vi "Get Category Summaries.vi"(8 "error in (no error)":errorcluster, 9 "Month":T1, 10 "YYYY":i32, 11 "Database in":refnum<class "Account History.lvclass">) -> (0 "error out":errorcluster, 2 "Category Summaries":refnum<class "Expense Summary.lvclass">[](array[class]), 3 "Database out":refnum<class "Account History.lvclass">)   [LabVIEW 2018, in "Account History.lvclass"]
uses:
  Account History.lvclass
  Expense Summary/Expense Summary.lvclass
  Month.ctl
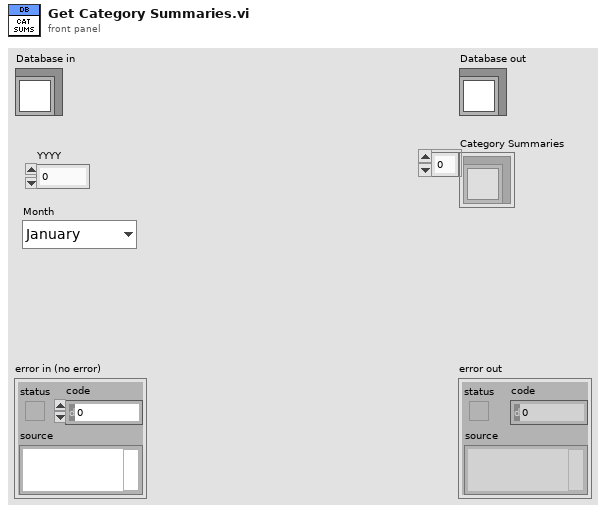
[diagram p1: front panel]
types:
  T1 = typedef "Account History.lvclass/Month.ctl" = enum16{"January", "February", "March", "April", "May", "June", "July", "August", "September", "October", "November", "December"}
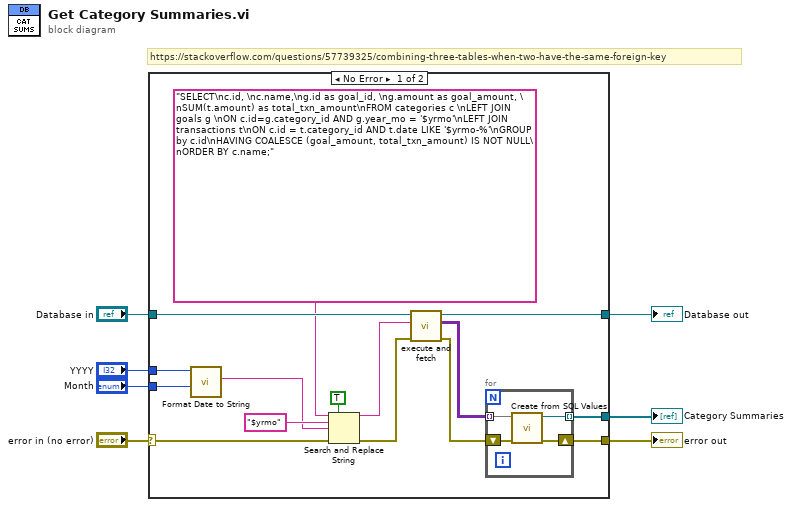
[diagram p0: block diagram]
diagram:
  # "https://stackoverflow.com/questions/57739325/combining-three-tables-when-two-have-the-same-foreign-key"
  n1 = case shown="No Error" "error in (no error)" {
    selector: "error in (no error)" -> [w17 w27]
    tunnel: [w20 w28] -> w7
    tunnel: "Database in" -> [w19 w28]
    tunnel: [w18 w27] -> w5
    tunnel: [w11 _] -> w3
    tunnel: "YYYY" -> [w9 _]
    tunnel: "Month" -> [w8 _]
    frame No Error {
      n2 = call "Format Date to String.vi"("Month"=w8, "YYYY"=w9) -> ("Year-Mo"=w10:string)  [unwired: 9 in]
      n3 = Search and Replace String(replace all?=TRUE ("replace all? (F)"), input string="SELECT\nc.id, \nc.name,\ng.id as goal_id, \ng.amount as goal_amount, \nSUM(t.amount) as total_txn_amount\nFROM categories c \nLEFT JOIN goals g \nON c.id=g.category_id AND g.year_mo = '$yrmo'\nLEFT JOIN transactions t\nON c.id = t.category_id AND t.date LIKE '$yrmo-%'\nGROUP by c.id\nHAVING COALESCE (goal_amount, total_txn_amount) IS NOT NULL\nORDER BY c.name;", search string="$yrmo", replace string=w10, error in=w17) -> (result string=w12:string, error out=w13:errorcluster)  [unwired: 3 in, 2 out]
      n4 = call "execute and fetch.vi"("error in (no error)"=w13, "SQL query"=w12, "Database in"=w19) -> ("error out"=w21:errorcluster, "recordset data"=w22:variant[][], "Database out"=w20:refnum<class "Account History.lvclass">)  [unwired: 5 in, 1 out]
      n5 = for {
        tunnel: w22 -> [w25] mode=indexing
        shift-right: [w23] -> w18
        shift-left: w21 -> [w26]
        tunnel: [w24] -> w11 mode=indexing
        n6 = call "Create from SQL Values.vi"("error in (no error)"=w26, "recordset data"=w25) -> ("error out"=w23:errorcluster, "Expense Summary out"=w24:refnum<class "Expense Summary.lvclass">)  [unwired: 8 in]
      }
    }
    frame Error {
    }
  }
  "error out" <- w5
  "Database out" <- w7
  "Category Summaries" <- w3
